vi "PLC_WriteData(U8).vi"(8 "error in (no error)":errorcluster, 9 "data":u8, 10 "LogicName":string, 11 "Message Enqueuer":refnum<class "Message Enqueuer.lvclass">) -> (0 "error out":errorcluster)   [LabVIEW 2025, in "PLC_API.lvlib"]
uses:
  PLC_API.lvlib
  <vilib>/ActorFramework/Message Enqueuer/Message Enqueuer.lvclass
  PLC_Module/PLC_Module Messages/WriteData Msg/WriteData Msg.lvclass/WriteData Msg.ctl
  <vilib>/ActorFramework/Message Enqueuer/Message Enqueuer.lvclass/Message Enqueuer.ctl
  <vilib>/ActorFramework/Message Enqueuer/Enqueue.vi
  PLC_Module/PLC_Module Messages/WriteData Msg/WriteData Msg.lvclass
  <vilib>/ActorFramework/Message Priority Queue/Priority Enqueue.vi
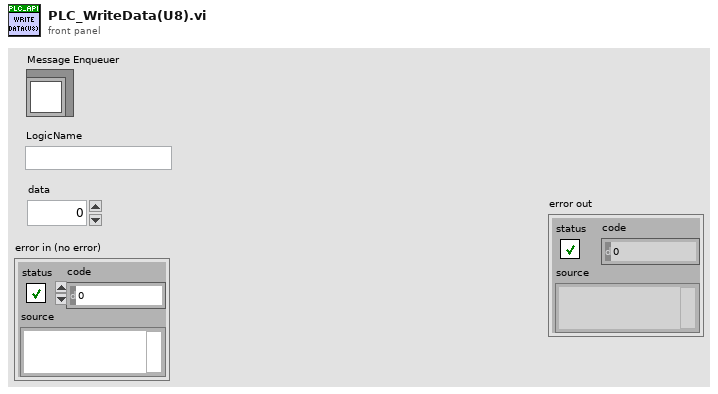
[diagram p1: front panel]
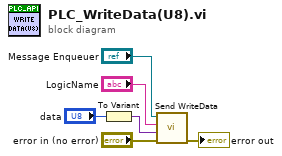
[diagram p0: block diagram]
diagram:
  n1 = To Variant(anything="data") -> (Variant=w1:variant)
  n2 = call "Send WriteData.vi"("error in (no error)"="error in (no error)", "Data"=w1, "LogicName"="LogicName", "Message Enqueuer"="Message Enqueuer") -> ("error out"=→"error out":errorcluster)  [unwired: 6 in, 1 out]
